vi "svx_Get Wav List.vi"(7 "name of the file":string, 8 "error in (no error)":errorcluster, 9 "target OS":T1(ring)=enum."Windows 95/NT") -> (0 "error out":errorcluster, 1 "example data folder":path, 2 "Path":path[](array[path]), 3 "file names":string[](array[string]), 4 "index":i32, 5 "appended path":path)   [LabVIEW 2017]
doc: "Obtains matching WAV files found at <LabVIEW>\\examples\\Sound and Vibration\\Example Data."
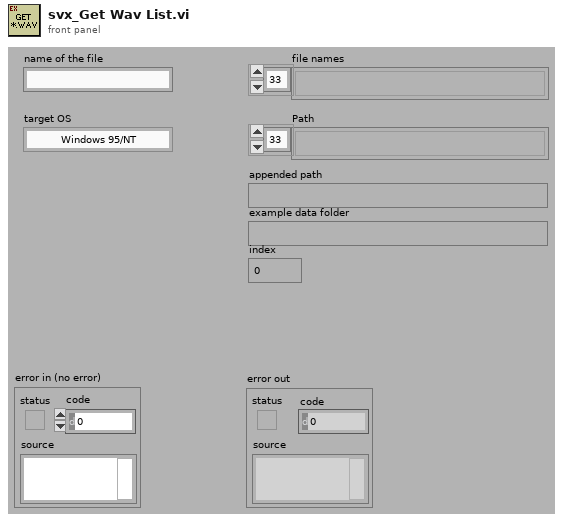
[diagram p1: front panel]
types:
  T1 = enum32{"invalid OS target", "Mac OS", "Windows 3.1", "Windows 95/NT", "Solaris 1", "Solaris 2", "HP-UX", "PowerMAX", "Linux", "Irix", "Rhapsody", "BeOS", "AIX", "OSF1", "VxWorks", "PharLap", "Carbon"}
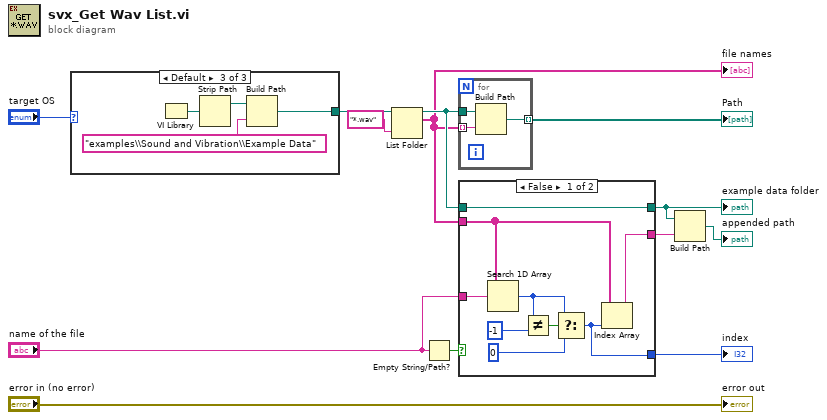
[diagram p0: block diagram]
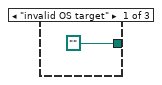
[diagram p2: hidden frame]
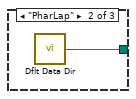
[diagram p3: hidden frame]
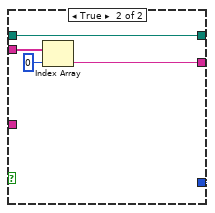
[diagram p4: hidden frame]
diagram:
  n1 = case shown="Default" "target OS" {
    tunnel: [path "" w15 w16] -> w12
    frame "invalid OS target" {
    }
    frame "PharLap" {
      n2 = call <vilib>:"Dflt Data Dir.vi"() -> ("App:Default Data Directory"=w15:path)
    }
    frame Default {
      n3 = VI Library() -> (path=w17:path)
      n4 = Strip Path(path=w17) -> (stripped path=w18:path)  [unwired: 1 out]
      n5 = Build Path(base path=w18, name or relative path="examples\\Sound and Vibration\\Example Data") -> (appended path=w16:path)
    }
  }
  n6 = List Folder(path=w12, pattern="*.wav") -> (path out=w7:path, filenames=w6:string[])  [unwired: 2 in, 2 out]
  "file names" <- w6
  n7 = Empty String/Path?(string/path="name of the file") -> (empty?=w9:bool)
  n8 = for {
    tunnel: [w22] -> w10 mode=indexing
    tunnel: w7 -> [w21]
    tunnel: w6 -> [w20] mode=indexing
    n9 = Build Path(base path=w21, name or relative path=w20) -> (appended path=w22:path)
  }
  "Path" <- w10
  n10 = case shown="False" w9 {
    tunnel: w6 -> [w27 w35]
    tunnel: "name of the file" -> [w31 _]
    tunnel: w7 -> [w30 w36]
    tunnel: [w30 w36] -> w4
    tunnel: [w24 w34] -> w5
    tunnel: [w23 0] -> w2
    frame False {
      n11 = Search 1D Array(1D array=w27, element=w31) -> (index of element=w25:i32)  [unwired: 1 in]
      n12 = Not Equal?(x=w25, y=-1) -> (x != y?=w28:bool)
      n13 = Select(t=w25, s=w28, f=0 ("Index")) -> (s? t:f=w23:i32)
      n14 = Index Array(array=w27, index=w23) -> (element=w24:string)
    }
    frame True {
      n15 = Index Array(array=w35, index=0 ("Index")) -> (element=w34:string)
    }
  }
  "example data folder" <- w4
  "index" <- w2
  n16 = Build Path(base path=w4, name or relative path=w5) -> (appended path=→"appended path":path)
  "error out" <- "error in (no error)"
